vi "Initialize.vi"(0 "VISA resource name":refnum<visa-resource-name>, 5 "ID Query (T: Check)":bool=TRUE, 7 "Reset (T: Reset)":bool=TRUE, 11 "error in (no error)":errorcluster) -> (4 "VISA resource name out":refnum<visa-resource-name>, 6 "idn string":string, 15 "error out":errorcluster {"code" format="%.0x"})   [LabVIEW 2013, in "Fluke 5XXX Series Multicalibrators.lvlib"]
doc: "This VI passes the addressing information in the instrument decriptor to the Instr Open VI and returns the instrument ID. You can optionally reset the instrument by setting the front panel reset control. You must run this VI before using any of the instrument driver VIs for this instrument."
uses:
  Fluke 5XXX Series Multicalibrators.lvlib
  <vilib>/Utility/error.llb/whitespace.ctl
panel:
  # "© 2005 National Instruments.  ALL RIGHTS RESERVED."
  # "Check\nDon't Check"
  # "Reset\nDon't Reset"
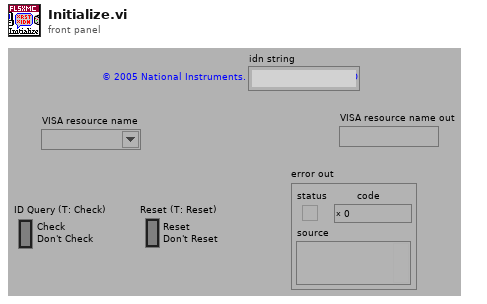
[diagram p1: front panel]
types:
  T1 = typedef "whitespace.ctl" = u16
  T2 = cluster{"Status":bool, "Code":i32, "Source (VI Name)":string}
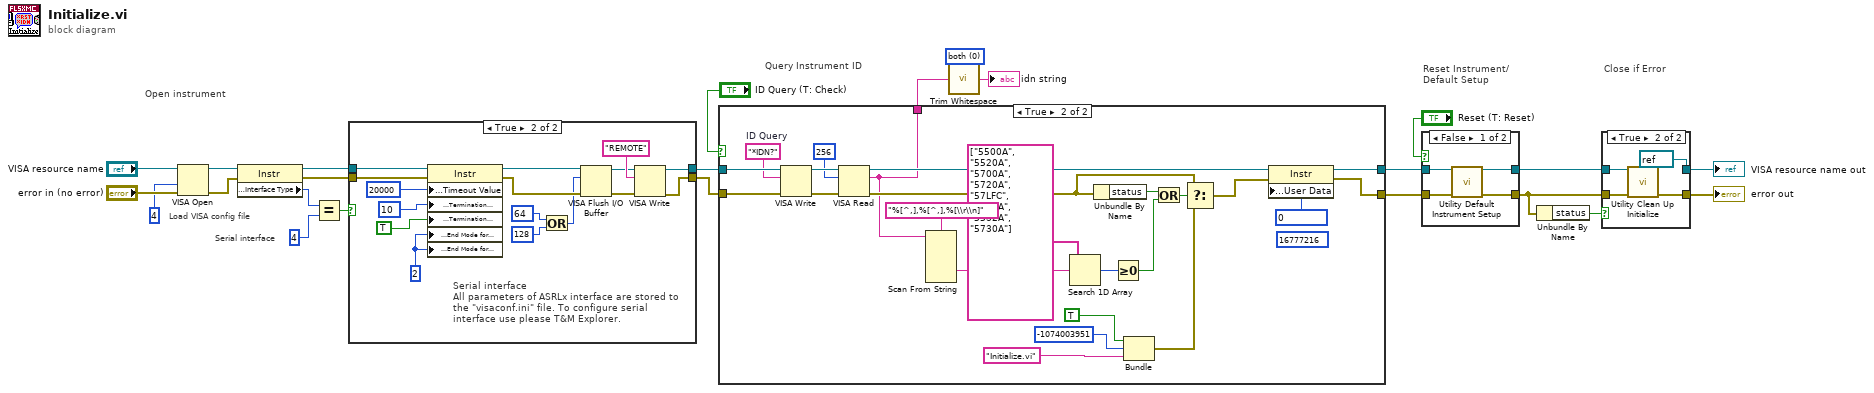
[diagram p0: block diagram]
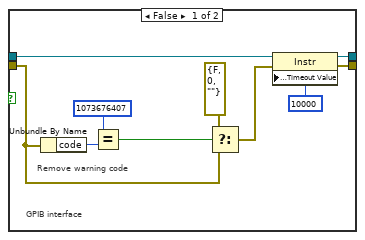
[diagram p2: hidden frame]
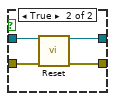
[diagram p4: hidden frame]
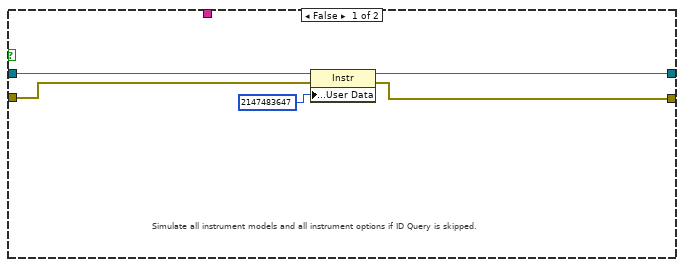
[diagram p5: hidden frame]
diagram:
  w2 = T1 0 items=["both", "start of string", "end of string"] ("location (both)")
  # "Serial interface"
  # "Load VISA config file"
  # "Close if Error"
  # "Query Instrument ID"
  # "Reset Instrument/\nDefault Setup"
  # "Open instrument"
  n1 = VISA Open(access mode=u32 4, error in (no error)="error in (no error)", VISA resource name="VISA resource name") -> (VISA resource name=w15:refnum<visa-resource-name>, error out=w14:errorcluster)  [unwired: 2 in]
  n2 = property class="Instr"(reference=w15, error in=w14) -> (reference out=w10:refnum<visa-resource-name>, error out=w11:errorcluster, "Interface Information:Interface Type"=w13:u16)
  n3 = Equal?(x=w13, y=u16 4) -> (x = y?=w12:bool)
  n4 = case shown="True" w12 {
    tunnel: w11 -> [w26 w49]
    tunnel: w10 -> [w34 w50]
    tunnel: [w33 w41] -> w6
    tunnel: [w32 w38] -> w5
    frame False {
      # "Remove warning code"
      # "GPIB interface"
      n5 = Unbundle By Name(w26) -> ("code"=w27:i32)
      n6 = Equal?(x=1073676407, y=w27) -> (x = y?=w29:bool)
      n7 = Select(t=errorcluster {"status"=FALSE, "code"=0, "source"=""} ("error out"), s=w29, f=w26) -> (s? t:f=w25:errorcluster)
      n8 = property class="Instr"(reference=w34, error in=w25, "General Settings:Timeout Value"=u32 10000 ("Tmo Value")) -> (reference out=w32:refnum<visa-resource-name>, error out=w33:errorcluster)
    }
    frame True {
      w45 = u16 2 ("ASRL End In")
      # "Serial interface\nAll parameters of ASRLx interface are stored to the \"visaconf.ini\" file. To configure serial interface use please T&M Explorer."
      n9 = property class="Instr"(reference=w50, error in=w49, "General Settings:Timeout Value"=u32 20000, "Message Based Settings:Termination Character"=u8 10 ("TermChar"), "Message Based Settings:Termination Character Enable"=TRUE ("TermChar En"), "Serial Settings:End Mode for Reads"=w45, "Serial Settings:End Mode for Writes"=w45) -> (reference out=w44:refnum<visa-resource-name>, error out=w43:errorcluster)
      n10 = Or(x=u32 64, y=u32 128) -> (x .or. y?=w35:u32)
      n11 = VISA Flush I/O Buffer(VISA resource name=w44, mask (16)=w35, error in (no error)=w43) -> (VISA resource name out=w39:refnum<visa-resource-name>, error out=w40:errorcluster)
      n12 = VISA Write(VISA resource name=w39, write buffer="REMOTE" ("ID Query"), error in (no error)=w40) -> (VISA resource name out=w38:refnum<visa-resource-name>, error out=w41:errorcluster)  [unwired: 1 out]
    }
  }
  n13 = case shown="True" "ID Query (T: Check)" {
    tunnel: [w54 w61] -> w23
    tunnel: [w55 w63] -> w24
    tunnel: w5 -> [w52 w78]
    tunnel: w6 -> [w53 w79]
    tunnel: [_ w56] -> w3
    frame False {
      # "Simulate all instrument models and all instrument options if ID Query is skipped."
      n14 = property class="Instr"(reference=w52, error in=w53, "General Settings:User Data"=u32 2147483647 ("y")) -> (reference out=w55:refnum<visa-resource-name>, error out=w54:errorcluster)
    }
    frame True {
      (unwired) u32 16777216 ("General Settings:User Data")
      w69 = "*IDN?"  # ID Query
      n15 = VISA Write(VISA resource name=w78, write buffer=w69, error in (no error)=w79) -> (VISA resource name out=w75:refnum<visa-resource-name>, error out=w73:errorcluster)  [unwired: 1 out]
      n16 = VISA Read(VISA resource name=w75, byte count=u32 256, error in (no error)=w73) -> (VISA resource name out=w64:refnum<visa-resource-name>, read buffer=w56:string, error out=w74:errorcluster)  [unwired: 1 out]
      n17 = Scan From String(format string="%[^,],%[^,],%[\\r\\n]" ("Format String"), input string=w56) -> (output 2=w58:string)  [unwired: 7 in, 3 out]
      n18 = Search 1D Array(1D array=string[] ["5500A", "5520A", "5700A", "5720A", "57LFC", "5522A", "5532A", "5730A"] ("Array Constant"), element=w58) -> (index of element=w57:i32)  [unwired: 1 in]
      n19 = Unbundle By Name(w74) -> ("status"=w71:bool)
      n20 = Greater Or Equal To 0?(x=w57) -> (x >= 0?=w76:bool)
      n21 = Bundle("Status"=TRUE, "Code"=-1074003951, "Source (VI Name)"="Initialize.vi") -> (w68:T2)  [unwired: 1 in]
      n22 = Or(x=w71, y=w76) -> (x .or. y?=w72:bool)
      n23 = Select(t=w74, s=w72, f=w68) -> (s? t:f=w62:T2)
      n24 = property class="Instr"(reference=w64, error in=w62, "General Settings:User Data"=u32 0) -> (reference out=w63:refnum<visa-resource-name>, error out=w61:errorcluster)
    }
  }
  n25 = call <vilib>:"Trim Whitespace.vi"("string"=w3, "location (both)"=w2) -> ("trimmed string"=→"idn string":string)
  n26 = case shown="False" "Reset (T: Reset)" {
    tunnel: w23 -> [w82 w84]
    tunnel: [w81 w87] -> w19
    tunnel: w24 -> [w83 w85]
    tunnel: [w80 w86] -> w18
    frame False {
      n27 = call "Utility Default Instrument Setup.vi"("VISA resource name"=w83, "error in (no error)"=w82) -> ("VISA resource name out"=w80:refnum<visa-resource-name>, "error out"=w81:errorcluster)  [unwired: 12 in]
    }
    frame True {
      n28 = call "Reset.vi"("VISA resource name"=w85, "error in (no error)"=w84) -> ("VISA resource name out"=w86:refnum<visa-resource-name>, "error out"=w87:errorcluster)  [unwired: 12 in]
    }
  }
  n29 = Unbundle By Name(w19) -> ("status"=w20:bool)
  n30 = case shown="True" w20 {
    tunnel: w18 -> [w89 w93]
    tunnel: w19 -> [w88 w92]
    tunnel: [w89 refnum<visa-resource-name> refnum ("VISA resource name out")] -> w17
    tunnel: [w88 w91] -> w16
    frame False {
    }
    frame True {
      n31 = call "Utility Clean Up Initialize.vi"("VISA session"=w93, "error in (no error)"=w92) -> ("error out"=w91:errorcluster)  [unwired: 13 in]
    }
  }
  "VISA resource name out" <- w17
  "error out" <- w16
